vi "Sub Process.vi"(8 "error in (no error)":errorcluster, 11 "Main Class in":refnum<class "Main Class.lvclass">) -> (0 "error out":errorcluster, 3 "Main Class out":refnum<class "Main Class.lvclass">)   [LabVIEW 2019, in "Main Class.lvclass"]
uses:
  Main Class.lvclass
  MPC_VirbVision/Ctrl/MainPage UI Ref_VirbVision.ctl
  Function/Main UI/Glb/Main_UI Gb.vi
  LLB/Commonly VI.lvlib
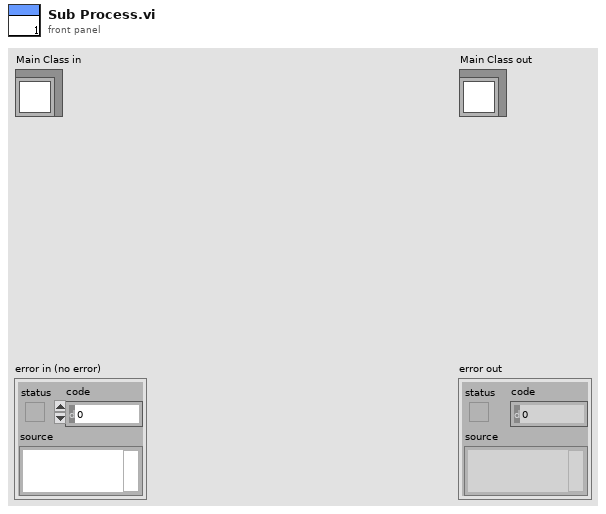
[diagram p1: front panel]
types:
  T1 = typedef "MainPage UI Ref_VirbVision.ctl" = cluster{"ProcessList":refnum<vi>, "Result Arr":refnum<vi>, "StopReceiveCmd":refnum<vi>}
  T2 = cluster{"ROI":string, "Numbers":i32, "Data":string[][]}[]
  T3 = cluster{"AutoRunFlg":refnum<vi>, "Action Finish Flg":refnum<vi>, "Remaining Action":refnum<vi>, "Btn_AutoRun":refnum<vi>, "Manual Flg":refnum<vi>, "Sub Process Error":refnum<vi>}
  T4 = typedef "SwitchBtn.ctl" = bool
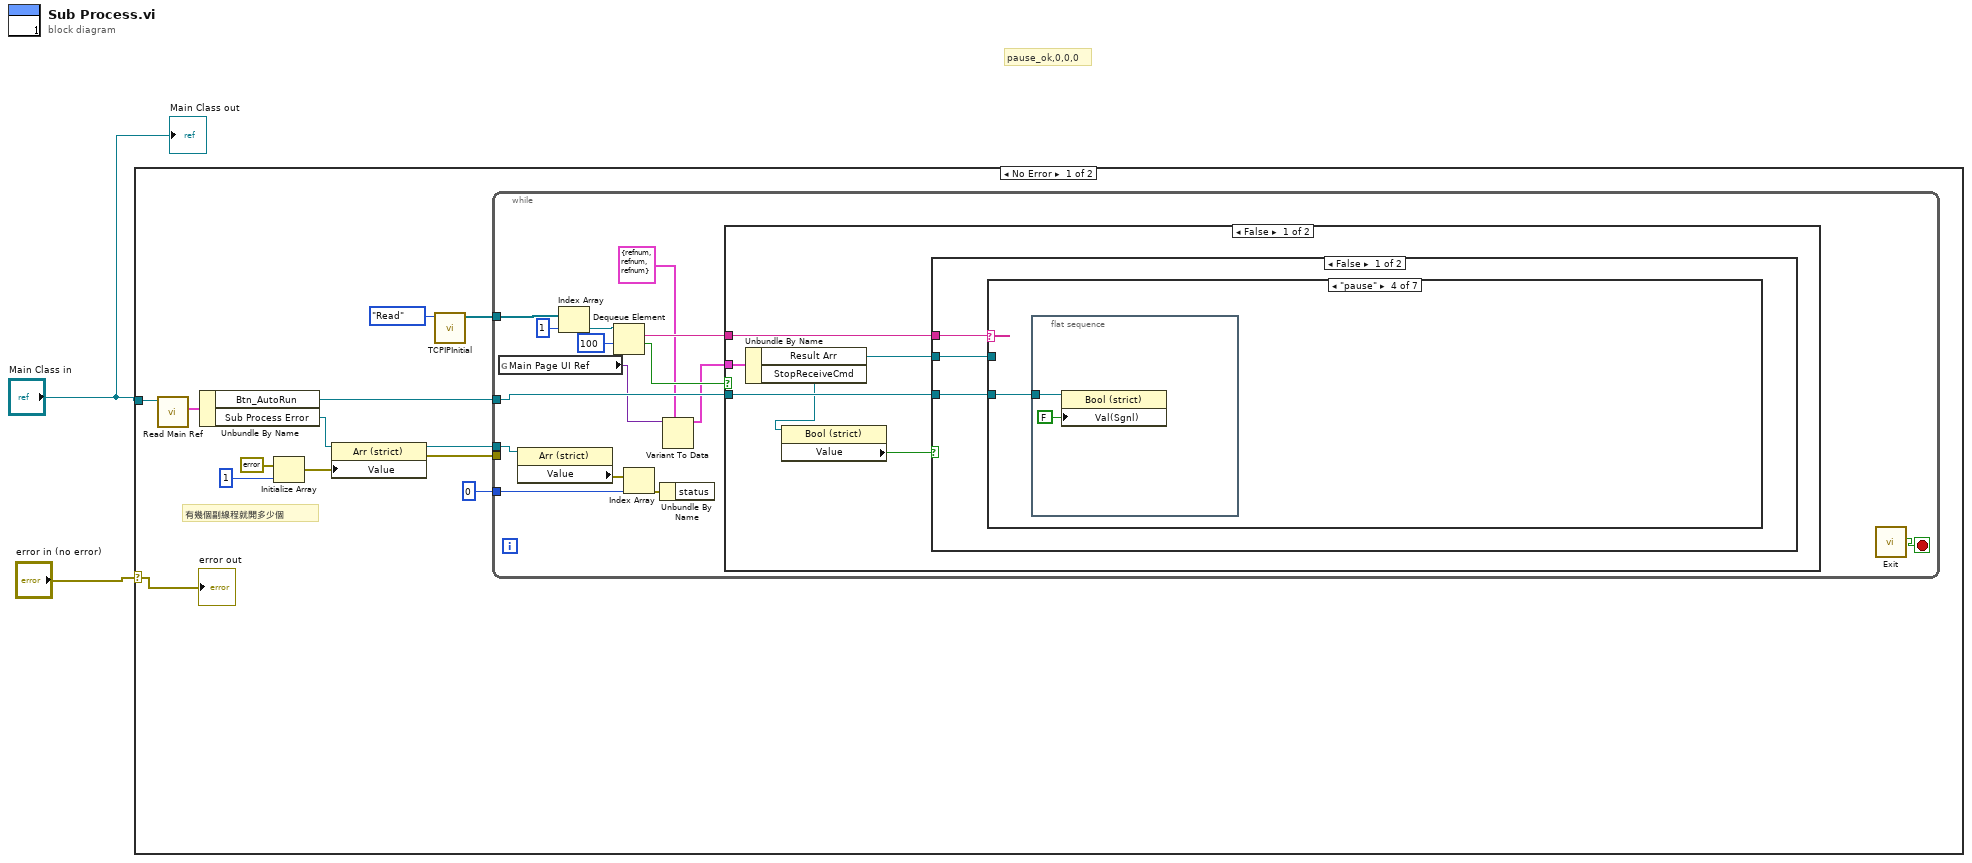
[diagram p0: block diagram]
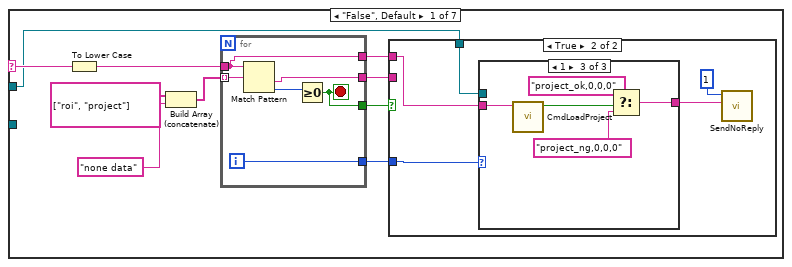
[diagram p2: hidden frame]
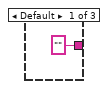
[diagram p4: hidden frame]
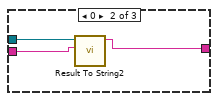
[diagram p5: hidden frame]
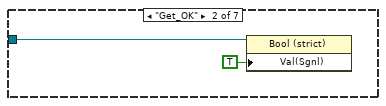
[diagram p6: hidden frame]
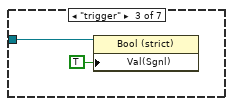
[diagram p7: hidden frame]
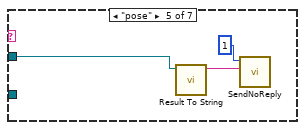
[diagram p8: hidden frame]
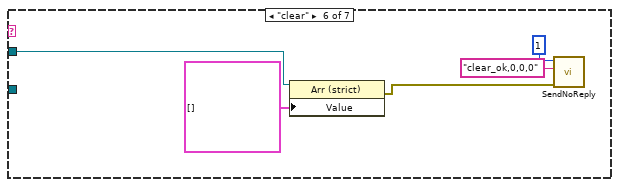
[diagram p9: hidden frame]
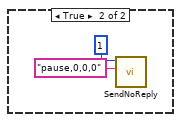
[diagram p11: hidden frame]
diagram:
  # "pause_ok,0,0,0"
  n1 = case shown="No Error" "error in (no error)" {
    selector: "error in (no error)" -> [w5 _]
    tunnel: "Main Class in" -> [w15 _]
    frame No Error {
      # "有幾個副線程就開多少個"
      n2 = call-dynamic "Read Main Ref.vi"("Main Process Class in"=w15) -> ("Main Ref"=w14:T3)  [unwired: 8 in, 2 out]
      n3 = Unbundle By Name(w14) -> ("Btn_AutoRun"=w13:refnum<vi>, "Sub Process Error"=w12:refnum<vi>)
      n4 = Initialize Array(errorcluster {"status"=FALSE, "code"=0, "source"=""} ("error"), 1 ("dimension size")) -> (w10:errorcluster[])
      n5 = property class="Arr (strict)"(reference=w12, "Value"=w10) -> (reference out=w7:refnum<vi>, error out=w8:errorcluster)  [unwired: 1 in]
      n6 = call "TCPIPInitial.vi"("Enum"=enum16{"initial", "Read", "release"}."Read") -> ("SN_Reply"=w3:refnum<queue>[])  [unwired: 7 in, 3 out]
      n7 = while {
        tunnel: w13 -> [w20]
        tunnel: w8 -> [_]
        tunnel: w7 -> [w30]
        tunnel: 0 -> [w28]
        tunnel: w3 -> [w25]
        stop <- w26 stop-if-true
        n8 = global read "Main_UI Gb.vi" "Main Page UI Ref"() -> (w16:variant)
        n9 = property class="Arr (strict)"(reference=w30) -> ("Value"=w29:errorcluster[])  [unwired: 1 in, 2 out]
        n10 = Index Array(array=w25, index=1) -> (element=w23:refnum<queue>)
        n11 = Dequeue Element(queue=w23, timeout in ms (-1)=100) -> (element=w22:string, timed out?=w19:bool)  [unwired: 1 in, 2 out]
        n12 = Index Array(array=w29, index=w28) -> (element=w27:errorcluster)
        n13 = Unbundle By Name(w27) -> ()  [unwired: 1 out]
        n14 = Variant To Data(type=T1 {"ProcessList"=refnum, "Result Arr"=refnum, "StopReceiveCmd"=refnum} ("Main Page UIRef"), Variant=w16) -> (data=w18:T1)  [unwired: 1 in, 1 out]
        n15 = case shown="False" w19 {
          tunnel: w22 -> [w36 _]
          tunnel: w20 -> [w35 _]
          tunnel: w18 -> [w34 _]
          frame False {
            n16 = Unbundle By Name(w34) -> ("Result Arr"=w33:refnum<vi>, "StopReceiveCmd"=w32:refnum<vi>)
            n17 = property class="Bool (strict)"(reference=w32) -> ("Value"=w31:T4)  [unwired: 1 in, 2 out]
            n18 = case shown="False" w31 {
              tunnel: w36 -> [w39 _]
              tunnel: w35 -> [w38 _]
              tunnel: w33 -> [w37 _]
              frame False {
                n19 = case shown="\"pause\"" w39 {
                  selector: w39 -> [w43 _ _ _ _ _ _]
                  tunnel: w38 -> [_ w71 w73 w74 _ _ _]
                  tunnel: w37 -> [w41 _ _ _ w79 w84 _]
                  frame "False", Default {
                    n20 = To Lower Case(string=w43) -> (all lower case string=w42:string)
                    n21 = Build Array (concatenate)(string[] ["roi", "project"], "none data") -> (w47:string[])
                    n22 = for {
                      tunnel: w42 -> [w65]
                      tunnel: w47 -> [w69] mode=indexing
                      tunnel: [w67] -> w44
                      tunnel: [w66] -> w46
                      tunnel: [w65] -> w45
                      tunnel: [w64] -> w40
                      i -> [w67]
                      stop <- w66 stop-if-true
                      n23 = Match Pattern(string=w65, regular expression=w69) -> (after substring=w64:string, offset past match=w68:i32)  [unwired: 1 in, 2 out]
                      n24 = Greater Or Equal To 0?(x=w68) -> (x >= 0?=w66:bool)
                    }
                    n25 = case shown="True" w46 {
                      tunnel: w45 -> [_ w52]
                      tunnel: w44 -> [_ w53]
                      tunnel: w41 -> [_ w54]
                      tunnel: w40 -> [_ _]
                      frame False {
                      }
                      frame True {
                        n26 = case shown="1" w53 {
                          tunnel: w54 -> [_ w58 _]
                          tunnel: w52 -> [_ w57 w63]
                          tunnel: ["" ("SendCmd") w56 w60] -> w51
                          frame Default {
                          }
                          frame 0 {
                            n27 = call "Result To String2.vi"("CmdName"=w57, "Result"=w58) -> ("SendCmd"=w56:string)  [unwired: 9 in]
                          }
                          frame 1 {
                            n28 = call "CmdLoadProject.vi"("String"=w63) -> ("loadok"=w62:bool)  [unwired: 10 in]
                            n29 = Select(t="project_ok,0,0,0", s=w62, f="project_ng,0,0,0") -> (s? t:f=w60:string)
                          }
                        }
                        n30 = call "SendNoReply.vi"("DataIn"=w51, "index"=1) -> ()  [unwired: 9 in, 1 out]
                      }
                    }
                  }
                  frame "Get_OK" {
                    n31 = property class="Bool (strict)"(reference=w71, "Val(Sgnl)"=TRUE ("Value (Signaling)")) -> ()  [unwired: 1 in, 2 out]
                  }
                  frame "trigger" {
                    n32 = property class="Bool (strict)"(reference=w73, "Val(Sgnl)"=TRUE ("Value (Signaling)")) -> ()  [unwired: 1 in, 2 out]
                  }
                  frame "pause" {
                    n33 = flat-sequence {
                      tunnel: w74 -> [w75]
                      frame #0 {
                        n34 = property class="Bool (strict)"(reference=w75, "Val(Sgnl)"=FALSE ("Value (Signaling)")) -> ()  [unwired: 1 in, 2 out]
                      }
                    }
                  }
                  frame "pose" {
                    n35 = call "Result To String.vi"("Result"=w79) -> ("SendCmd"=w77:string)  [unwired: 10 in]
                    n36 = call "SendNoReply.vi"("DataIn"=w77, "index"=1) -> ()  [unwired: 9 in, 1 out]
                  }
                  frame "clear" {
                    n37 = property class="Arr (strict)"(reference=w84, "Value"=T2 []) -> (error out=w81:errorcluster)  [unwired: 1 in, 1 out]
                    n38 = call "SendNoReply.vi"("error in (no error)"=w81, "DataIn"="clear_ok,0,0,0", "index"=1) -> ()  [unwired: 8 in, 1 out]
                  }
                  frame "getall" {
                  }
                }
              }
              frame True {
                n39 = call "SendNoReply.vi"("DataIn"="pause,0,0,0", "index"=1) -> ()  [unwired: 9 in, 1 out]
              }
            }
          }
          frame True {
          }
        }
        n40 = call "Exit.vi"() -> ("ExitOut"=w26:bool)  [unwired: 11 in]
      }
      "error out" <- w5
    }
    frame Error {
    }
  }
  "Main Class out" <- "Main Class in"
